vi "read.vi"(8 "error in (no error)":errorcluster, 9 "Timeout":i32=25000, 10 "NumberOfBytes":i32, 11 "M1M3SAL in":refnum<class "M1M3SAL.lvclass">) -> (0 "error out":errorcluster, 2 "Data":u8[](array[numeric]), 3 "M1M3SAL out":refnum<class "M1M3SAL.lvclass">)   [LabVIEW 2016, in "M1M3SAL.lvlib" / "M1M3SAL.lvclass"]
uses:
  M1M3SAL.lvclass
  M1M3SAL.lvclass/M1M3SAL.ctl
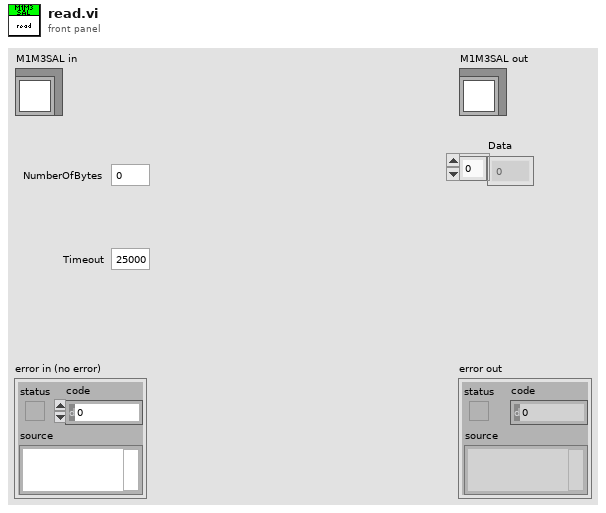
[diagram p1: front panel]
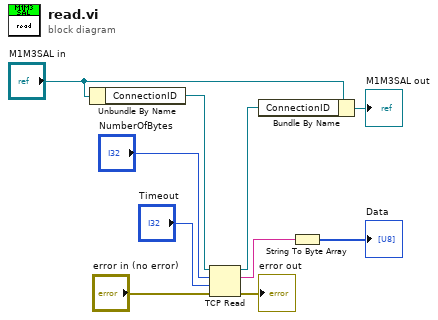
[diagram p0: block diagram]
diagram:
  n1 = Unbundle By Name("M1M3SAL in") -> ("ConnectionID"=w8:refnum<k5>)
  n2 = TCP Read(connection ID=w8, bytes to read="NumberOfBytes", error in (no error)="error in (no error)", 9:"Timeout") -> (connection ID out=w7:refnum<k5>, data out=w5:string, error out=→"error out":errorcluster)  [unwired: 1 in]
  n3 = Bundle By Name(cluster="M1M3SAL in", "ConnectionID"=w7) -> (→"M1M3SAL out":refnum<class "M1M3SAL.lvclass">)
  n4 = String To Byte Array(string=w5) -> (unsigned byte array=→"Data":u8[])
